vi "ClimbBegin.vi"(8 "error in (no error)":errorcluster) -> (0 "error out":errorcluster)   [LabVIEW 2023]
uses:
  <vilib>/Rock Robotics/WPI/ThirdParty/REV Robotics/REVLib/Typedef/Spark MAX Sensor Type.ctl
  <vilib>/Rock Robotics/WPI/ThirdParty/REV Robotics/REVLib/Typedef/Spark MAX Limit Switch Polarity.ctl
  <vilib>/Rock Robotics/WPI/ThirdParty/REV Robotics/REVLib/Typedef/Spark MAX Limit Direction.ctl
  <vilib>/Rock Robotics/WPI/ThirdParty/REV Robotics/REVLib/Typedef/Spark MAX Idle Mode.ctl
  <vilib>/Rock Robotics/WPI/ThirdParty/REV Robotics/REVLib/Typedef/Spark MAX Motor Type.ctl
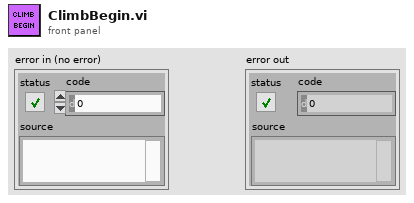
[diagram p1: front panel]
types:
  T1 = typedef "Spark MAX Sensor Type.ctl" = enum16{"No Sensor", "Hall Sensor", "Encoder", "-Not Available-", "Analog", "Alternate Encoder", "Duty Cycle"}
  T2 = typedef "Spark MAX Limit Switch Polarity.ctl" = enum16{"Normally Open", "Normally Closed"}
  T3 = typedef "Spark MAX Limit Direction.ctl" = enum16{"Forward Limit", "Reverse Limit"}
  T4 = typedef "Spark MAX Idle Mode.ctl" = enum16{"Coast", "Brake"}
  T5 = typedef "Spark MAX Motor Type.ctl" = enum16{"Brushed", "Brushless"}
  T6 = typedef "WPI_MotorControlDeviceRef.ctl" = cluster{"DeviceStatus":errorcluster, "Type":T7, "PWM":cluster{"PWM Channel":T8, "DeadBand":T9}, "CAN":cluster{"Device Number":u8, "SetOutput VI Ref":variant, "GetOutput VI Ref":variant, "Enable VI Ref":variant, "Disable VI Ref":variant, "Data":variant}, "Invert":bool, "DIO PWM":cluster{"PWM \"Enable\" Channel":T8, "DIOChannel":T10, "PWM Rate":dbl}}
  T7 = typedef "WPI_MotorControlType.ctl" = enum16{"PWM", "CAN", "DIO PWM"}
  T8 = typedef "FPGA_DIOPWMChannel.ctl" = enum8{"PWM 0", "PWM 1", "PWM 2", "PWM 3", "PWM 4", "PWM 5", "PWM 6", "PWM 7", "PWM 8", "PWM 9", "PWM MXP 0", "PWM MXP 1", "PWM MXP 2", "PWM MXP 3", "PWM MXP 4", "PWM MXP 5", "PWM MXP 6", "PWM MXP 7", "PWM MXP 8", "PWM MXP 9", "Invalid"}
  T9 = typedef "WPI_PWMDeadband.ctl" = cluster{"Name":string, "maxPositivePwm":i32, "minPositivePwm":i32, "centerPwm":i32, "maxNegativePwm":i32, "minNegativePwm":i32, "angularRange":u16}
  T10 = typedef "FPGA_DIOChannel.ctl" = enum8{"DIO 0", "DIO 1", "DIO 2", "DIO 3", "DIO 4", "DIO 5", "DIO 6", "DIO 7", "DIO 8", "DIO 9", "DIO MXP 0", "DIO MXP 1", "DIO MXP 2", "DIO MXP 3", "DIO MXP 4", "DIO MXP 5", "DIO MXP 6", "DIO MXP 7", "DIO MXP 8", "DIO MXP 9", "DIO MXP 10", "DIO MXP 11", "DIO MXP 12", "DIO MXP 13", "DIO MXP 14", "DIO MXP 15", "SPI Port CS1", "SPI Port CS2", "SPI Port CS3", "SPI Port MISO", "SPI Port MOSI", "Invalid"}
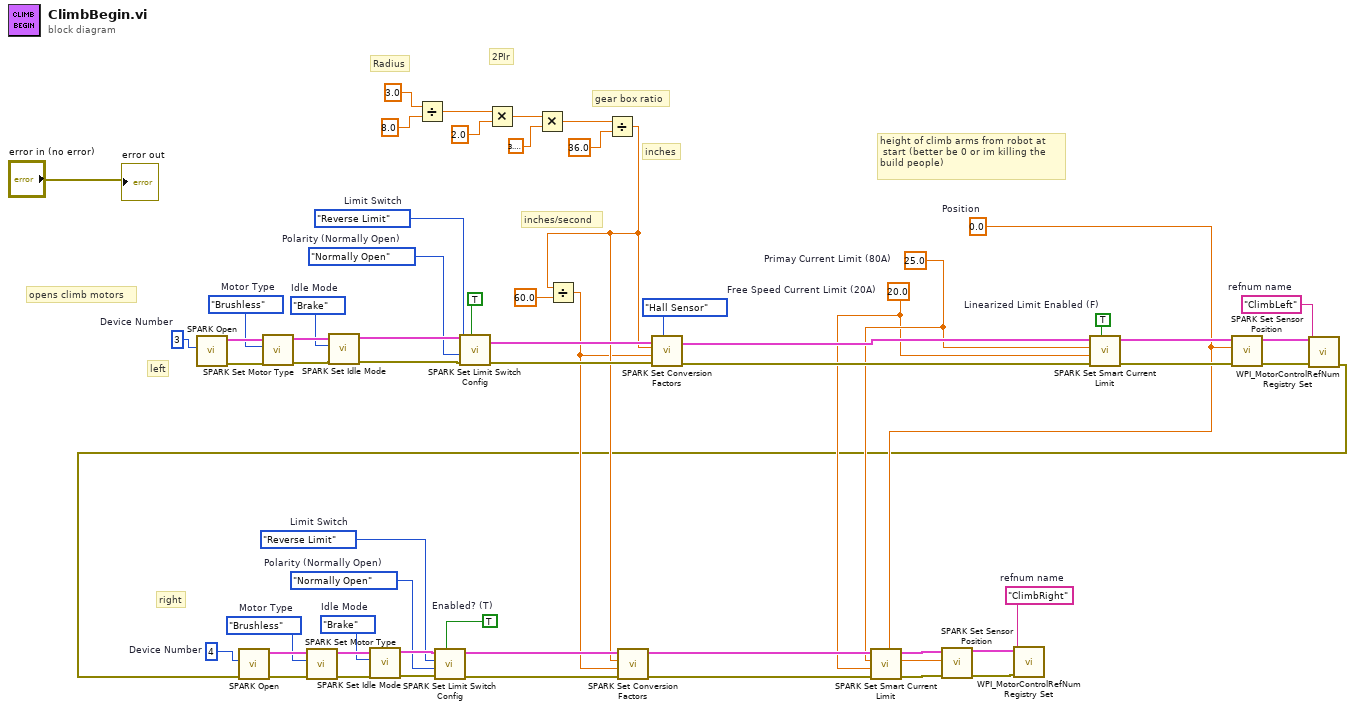
[diagram p0: block diagram]
diagram:
  w1 = TRUE  # Linearized Limit Enabled (F)
  w9 = 0.0  # Position
  w27 = TRUE  # Enabled? (T)
  w4 = 20.0  # Free Speed Current Limit (20A)
  w5 = 25.0  # Primay Current Limit (80A)
  w29 = Spark_MAX_Limit_Switch_Polarity."Normally Open"  # Polarity (Normally Open)
  w30 = Spark_MAX_Limit_Direction."Reverse Limit"  # Limit Switch
  w31 = Spark_MAX_Limit_Switch_Polarity."Normally Open"  # Polarity (Normally Open)
  w32 = Spark_MAX_Limit_Direction."Reverse Limit"  # Limit Switch
  w42 = Spark_MAX_Idle_Mode."Brake"  # Idle Mode
  w43 = Spark_MAX_Idle_Mode."Brake"  # Idle Mode
  w46 = Spark_MAX_Motor_Type."Brushless"  # Motor Type
  w47 = Spark_MAX_Motor_Type."Brushless"  # Motor Type
  w48 = "ClimbRight"  # refnum name
  w49 = "ClimbLeft"  # refnum name
  w53 = u8 4  # Device Number
  w54 = u8 3  # Device Number
  # "inches/second"
  # "inches"
  # "height of climb arms from robot at\n start (better be 0 or im killing the \nbuild people)"
  # "gear box ratio"
  # "2PIr"
  # "Radius"
  # "opens climb motors"
  # "right"
  # "left"
  n1 = call <vilib>:"SPARK Open.vi"("Device Number"=w54) -> ("error out"=w55:errorcluster, "MotorControlDeviceRef"=w56:T6)  [unwired: 9 in]
  n2 = call <vilib>:"SPARK Set Motor Type.vi"("error in (no error)"=w55, "Motor Type"=w47, "MotorControlDevRef"=w56) -> ("error out"=w41:errorcluster, "MotorControlDeviceRef"=w45:T6)  [unwired: 7 in]
  n3 = call <vilib>:"SPARK Set Idle Mode.vi"("error in (no error)"=w41, "Idle Mode"=w42, "MotorControlDeviceRef in"=w45) -> ("error out"=w33:errorcluster, "MotorControlDeviceRef out"=w34:T6)  [unwired: 7 in]
  n4 = Divide(x=3.0, y=8.0) -> (x/y=w19:dbl)
  n5 = call <vilib>:"SPARK Set Limit Switch Config.vi"("Enabled? (T)"=TRUE, "error in (no error)"=w33, "Polarity (Normally Open)"=w31, "Limit Switch"=w32, "MotorControlDeviceRef in"=w34) -> ("error out"=w24:errorcluster, "MotorControlDeviceRef out"=w26:T6)  [unwired: 5 in]
  n6 = Multiply(x=w19, y=2.0) -> (x*y=w17:dbl)
  n7 = Multiply(x=w17, y=3.141592653589793) -> (x*y=w15:dbl)
  n8 = Divide(x=w15, y=36.0) -> (x/y=w7:dbl)
  n9 = Divide(x=w7, y=60.0) -> (x/y=w6:dbl)
  n10 = call <vilib>:"SPARK Set Conversion Factors.vi"("Sensor Type (Hall Sensor)"=Spark_MAX_Sensor_Type."Hall Sensor", "error in (no error)"=w24, "Velocity Factor (1)"=w6, "Position Factor (1)"=w7, "MotorControlDeviceRef in"=w26) -> ("error out"=w23:errorcluster, "MotorControlDeviceRef out"=w25:T6)  [unwired: 5 in]
  n11 = call <vilib>:"SPARK Set Smart Current Limit.vi"("Linearized Limit Enabled (F)"=w1, "error in (no error)"=w23, "Free Speed Current Limit (20A)"=w4, "Primay Current Limit (80A)"=w5, "MotorControlDeviceRef in"=w25) -> ("error out"=w60:errorcluster, "MotorControlDeviceRef out"=w59:T6)  [unwired: 5 in]
  n12 = call <vilib>:"SPARK Set Sensor Position.vi"("error in"=w60, "Position"=w9, "MotorControlDeviceRef"=w59) -> ("error out"=w40:errorcluster, "MotorControlDeviceRef"=w51:T6)  [unwired: 7 in]
  n13 = call <vilib>:"WPI_MotorControlRefNum Registry Set.vi"("error in (no error)"=w40, "refnum name"=w49, "MotorControlDevRef"=w51) -> ("error out"=w2:errorcluster)  [unwired: 7 in, 1 out]
  n14 = call <vilib>:"SPARK Open.vi"("error in (no error)"=w2, "Device Number"=w53) -> ("error out"=w39:errorcluster, "MotorControlDeviceRef"=w52:T6)  [unwired: 8 in]
  n15 = call <vilib>:"SPARK Set Motor Type.vi"("error in (no error)"=w39, "Motor Type"=w46, "MotorControlDevRef"=w52) -> ("error out"=w38:errorcluster, "MotorControlDeviceRef"=w44:T6)  [unwired: 7 in]
  n16 = call <vilib>:"SPARK Set Idle Mode.vi"("error in (no error)"=w38, "Idle Mode"=w43, "MotorControlDeviceRef in"=w44) -> ("error out"=w35:errorcluster, "MotorControlDeviceRef out"=w36:T6)  [unwired: 7 in]
  n17 = call <vilib>:"SPARK Set Limit Switch Config.vi"("Enabled? (T)"=w27, "error in (no error)"=w35, "Polarity (Normally Open)"=w29, "Limit Switch"=w30, "MotorControlDeviceRef in"=w36) -> ("error out"=w11:errorcluster, "MotorControlDeviceRef out"=w13:T6)  [unwired: 5 in]
  n18 = call <vilib>:"SPARK Set Conversion Factors.vi"("error in (no error)"=w11, "Velocity Factor (1)"=w6, "Position Factor (1)"=w7, "MotorControlDeviceRef in"=w13) -> ("error out"=w10:errorcluster, "MotorControlDeviceRef out"=w12:T6)  [unwired: 6 in]
  n19 = call <vilib>:"SPARK Set Smart Current Limit.vi"("error in (no error)"=w10, "Free Speed Current Limit (20A)"=w4, "Primay Current Limit (80A)"=w5, "MotorControlDeviceRef in"=w12) -> ("error out"=w58:errorcluster, "MotorControlDeviceRef out"=w57:T6)  [unwired: 6 in]
  n20 = call <vilib>:"SPARK Set Sensor Position.vi"("error in"=w58, "Position"=w9, "MotorControlDeviceRef"=w57) -> ("error out"=w37:errorcluster, "MotorControlDeviceRef"=w50:T6)  [unwired: 7 in]
  n21 = call <vilib>:"WPI_MotorControlRefNum Registry Set.vi"("error in (no error)"=w37, "refnum name"=w48, "MotorControlDevRef"=w50) -> ()  [unwired: 7 in, 2 out]
  "error out" <- "error in (no error)"
